vi "Format DescribeTagsResult_LVXML_TagSet.vi"(8 "error in (no error)":errorcluster, 11 "xmlDataIn":T4) -> (0 "error IO":errorcluster, 3 "DescribeTagsResponse":T1)   [LabVIEW 2014, in "AWS_EC2.lvlib" / "AWS_EC2.lvclass"]
uses:
  AWS_EC2.lvclass
  lv-xml-parser/r0/trunk/VI Source/EventType.ctl
  Response Typedefs/DescribeTagsResult.ctl
  EC2 Datatypes/TagSetItemType.ctl
  AWS_EC2.lvlib
  lv-xml-parser/r0/trunk/VI Source/LV XML Parser.lvlib
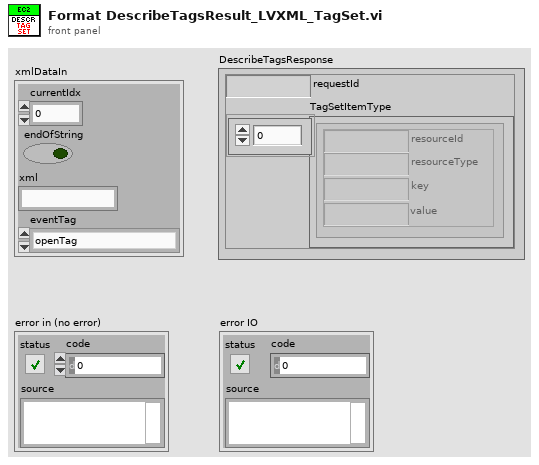
[diagram p1: front panel]
types:
  T1 = typedef "AWS_EC2.lvlib/DescribeTagsResult.ctl" = cluster{"requestId":string, "TagSetItemType":T2}
  T2 = typedef "AWS_EC2.lvlib/TagSetItemType.ctl" = cluster{"resourceId":string, "resourceType":string, "key":string, "value":string}[]
  T3 = typedef "LV XML Parser.lvlib/EventType.ctl" = enum16{"openTag", "endOpenTag", "closeTag", "comment", "endComment", "endOfFile", "attribute", "startXml"}
  T4 = cluster{"currentIdx":i32, "endOfString":bool, "xml":string, "eventTag":T3}
  T5 = cluster{"namespaceUri":string, "localName":string}
  T6 = cluster{"Attributes":cluster{"localName":string, "namespaceUri":string, "value":string}[], "localName":string, "namespaceUri":string, "valueXmlData":cluster{"currentIdx":i32, "endOfString":bool, "xml":string, "eventTag":T3}}[]
  T7 = cluster{"resourceId":string, "resourceType":string, "key":string, "value":string}[]
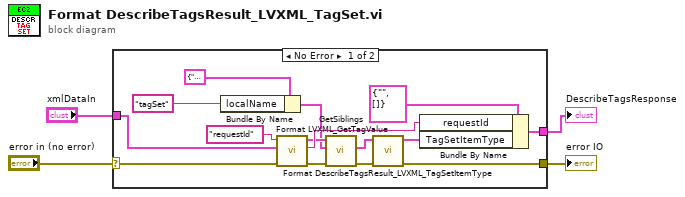
[diagram p0: block diagram]
diagram:
  n1 = case shown="No Error" "error in (no error)" {
    selector: "error in (no error)" -> [w5 w20]
    tunnel: "xmlDataIn" -> [w15 _]
    tunnel: [w13 _] -> w3
    tunnel: [w9 w20] -> w2
    frame No Error {
      n2 = Bundle By Name(cluster=T5 {"namespaceUri"="", "localName"=""} ("limitToTag"), "localName"="tagSet" ("Tag name")) -> (w11:T5)
      n3 = call "Format LVXML_GetTagValue.vi"("error in (no error)"=w5, "xmlDataIn"=w15, "Tag name"="requestId") -> ("error out"=w10:errorcluster, "Value"=w19:string, "xmlDataOut"=w12:T4)  [unwired: 6 in]
      n4 = call "GetSiblings.vi"("error in (no error)"=w10, "limitToTag"=w11, "xmlData"=w12) -> ("error out"=w6:errorcluster, "Siblings"=w7:T6)  [unwired: 7 in]
      n5 = call "Format DescribeTagsResult_LVXML_TagSetItemType.vi"("error in (no error)"=w6, "Siblings"=w7) -> ("error out"=w9:errorcluster, "Array"=w8:T7)  [unwired: 8 in]
      n6 = Bundle By Name(cluster=T1 {"requestId"="", "TagSetItemType"=[]} ("DescribeTagsResponse"), "requestId"=w19, "TagSetItemType"=w8) -> (w13:T1)
    }
    frame Error {
    }
  }
  "DescribeTagsResponse" <- w3
  "error IO" <- w2
